vi "Clousure.vi"(8 "error in (no error)":errorcluster, 11 "ConcreteProductA in":refnum<class "ConcreteProductA.lvclass">) -> (0 "error out":errorcluster, 3 "ConcreteProductA out":refnum<class "ConcreteProductA.lvclass">)   [LabVIEW 2020, in "FactoryMethod.lvlib" / "ConcreteProductA.lvclass"]
uses:
  ConcreteProductA.lvclass
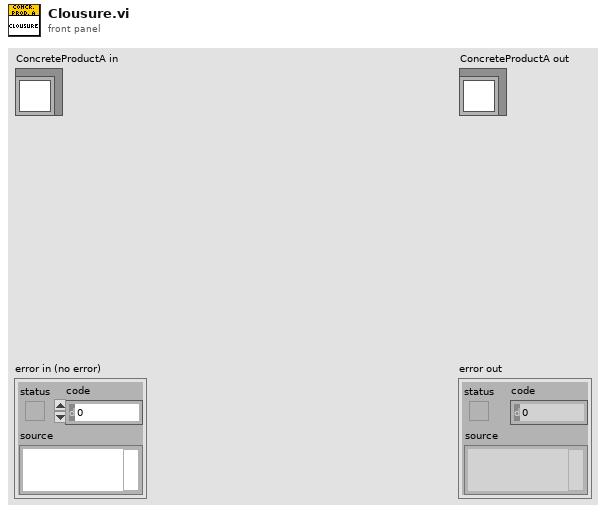
[diagram p1: front panel]
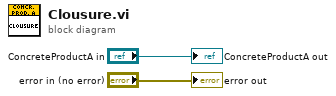
[diagram p0: block diagram]
diagram:
  "error out" <- "error in (no error)"
  "ConcreteProductA out" <- "ConcreteProductA in"
